vi "main.vi"() -> ()   [LabVIEW 2023] (continued)
      2445  18F106A7   00000004    8        00\tF7\tFF\tFF\tFF\tFF\tFF\tA1\r\n      2445  0CF104A7   00000004    8        F0\t60\t22\tFC\tFF\tFF\tFF\t50\r\n      2444  0CF103A7   00000004    8        17\t1F\t08\t60\tB1\t1F\t08\t50\r\n      2444  0CF102A7   00000004    8        30\t75\tE0\t2E\t80\tFF\tFF\tFD\r\n      2443  0C3C4D4A   00000004    8        BE\tFF\tFF\t7F\t18\tFF\tFF\t50\r\n      2443  0CF101A7   00000004    8        68\t00\t97\tCC\t00\t16\t39\t94\r\n      2442  18F120F0   00000004    8        2B\t75\t60\tB1\tB0\t01\tFF\tFF\r\n      2441  18F11FF0   00000004    8        FF\t3F\t90\t68\t88\t1B\t10\t0C\r\n      2462  1FFFFFFF   00000004    8        00\t20\tFF\tFF\tFF\tFF\tFF\tFF\r\n      2452  1FFFFFFF   00000004    8        00\t20\tFF\tFF\tFF\tFF\tFF\tFF\r\n      2447  1FFFFFFF   00000004    8        00\t20\tFF\tFF\tFF\tFF\tFF\tFF\r\n      2446  18F121F0   00000004    8        09\t19\t00\t00\tFF\tFF\tB0\t01\r\n      2445  18F106A7   00000004    8        00\tF7\tFF\tFF\tFF\tFF\tFF\tA1\r\n      2445  0CF104A7   00000004    8        F0\t60\t22\tFC\tFF\tFF\tFF\t50\r\n      2444  0CF103A7   00000004    8        17\t1F\t08\t60\tB1\t1F\t08\t50\r\n      2444  0CF102A7   00000004    8        30\t75\tE0\t2E\t80\tFF\tFF\tFD\r\n      2443  0C3C4D4A   00000004    8        BE\tFF\tFF\t7F\t18\tFF\tFF\t50\r\n      2443  0CF101A7   00000004    8        68\t00\t97\tCC\t00\t16\t39\t94\r\n      2442  18F120F0   00000004    8        2B\t75\t60\tB1\tB0\t01\tFF\tFF\r\n      2463  0CF101A7   00000004    8        68\t00\t97\tCC\t00\t16\t39\t95\r\n      2462  1FFFFFFF   00000004    8        00\t20\tFF\tFF\tFF\tFF\tFF\tFF\r\n      2452  1FFFFFFF   00000004    8        00\t20\tFF\tFF\tFF\tFF\tFF\tFF\r\n      2447  1FFFFFFF   00000004    8        00\t20\tFF\tFF\tFF\tFF\tFF\tFF\r\n      2446  18F121F0   00000004    8        09\t19\t00\t00\tFF\tFF\tB0\t01\r\n      2445  18F106A7   00000004    8        00\tF7\tFF\tFF\tFF\tFF\tFF\tA1\r\n      2445  0CF104A7   00000004    8        F0\t60\t22\tFC\tFF\tFF\tFF\t50\r\n      2444  0CF103A7   00000004    8        17\t1F\t08\t60\tB1\t1F\t08\t50\r\n      2444  0CF102A7   00000004    8        30\t75\tE0\t2E\t80\tFF\tFF\tFD\r\n      2443  0C3C4D4A   00000004    8        BE\tFF\tFF\t7F\t18\tFF\tFF\t50\r\n      2443  0CF101A7   00000004    8        68\t00\t97\tCC\t00\t16\t39\t94\r\n      2463  0CF102A7   00000004    8        30\t75\tE0\t2E\t80\tFF\tFF\tFD\r\n      2463  0CF101A7   00000004    8        68\t00\t97\tCC\t00\t16\t39\t95\r\n      2462  1FFFFFFF   00000004    8        00\t20\tFF\tFF\tFF\tFF\tFF\tFF\r\n      2452  1FFFFFFF   00000004    8        00\t20\tFF\tFF\tFF\tFF\tFF\tFF\r\n      2447  1FFFFFFF   00000004    8        00\t20\tFF\tFF\tFF\tFF\tFF\tFF\r\n      2446  18F121F0   00000004    8        09\t19\t00\t00\tFF\tFF\tB0\t01\r\n      2445  18F106A7   00000004    8        00\tF7\tFF\tFF\tFF\tFF\tFF\tA1\r\n      2445  0CF104A7   00000004    8        F0\t60\t22\tFC\tFF\tFF\tFF\t50\r\n      2444  0CF103A7   00000004    8        17\t1F\t08\t60\tB1\t1F\t08\t50\r\n      2444  0CF102A7   00000004    8        30\t75\tE0\t2E\t80\tFF\tFF\tFD\r\n      2443  0C3C4D4A   00000004    8        BE\tFF\tFF\t7F\t18\tFF\tFF\t50\r\n      2472  1FFFFFFF   00000004    8        00\t20\tFF\tFF\tFF\tFF\tFF\tFF\r\n      2463  0CF102A7   00000004    8        30\t75\tE0\t2E\t80\tFF\tFF\tFD\r\n      2463  0CF101A7   00000004    8        68\t00\t97\tCC\t00\t16\t39\t95\r\n      2462  1FFFFFFF   00000004    8        00\t20\tFF\tFF\tFF\tFF\tFF\tFF\r\n      2452  1FFFFFFF   00000004    8        00\t20\tFF\tFF\tFF\tFF\tFF\tFF\r\n      2447  1FFFFFFF   00000004    8        00\t20\tFF\tFF\tFF\tFF\tFF\tFF\r\n      2446  18F121F0   00000004    8        09\t19\t00\t00\tFF\tFF\tB0\t01\r\n      2445  18F106A7   00000004    8        00\tF7\tFF\tFF\tFF\tFF\tFF\tA1\r\n      2445  0CF104A7   00000004    8        F0\t60\t22\tFC\tFF\tFF\tFF\t50\r\n      2444  0CF103A7   00000004    8        17\t1F\t08\t60\tB1\t1F\t08\t50\r\n      2444  0CF102A7   00000004    8        30\t75\tE0\t2E\t80\tFF\tFF\tFD\r\n      2482  1FFFFFFF   00000004    8        00\t00\tFF\tFF\tFF\tFF\tFF\tFF\r\n      2472  1FFFFFFF   00000004    8        00\t20\tFF\tFF\tFF\tFF\tFF\tFF\r\n      2463  0CF102A7   00000004    8        30\t75\tE0\t2E\t80\tFF\tFF\tFD\r\n      2463  0CF101A7   00000004    8        68\t00\t97\tCC\t00\t16\t39\t95\r\n      2462  1FFFFFFF   00000004    8        00\t20\tFF\tFF\tFF\tFF\tFF\tFF\r\n      2452  1FFFFFFF   00000004    8        00\t20\tFF\tFF\tFF\tFF\tFF\tFF\r\n      2447  1FFFFFFF   00000004    8        00\t20\tFF\tFF\tFF\tFF\tFF\tFF\r\n      2446  18F121F0   00000004    8        09\t19\t00\t00\tFF\tFF\tB0\t01\r\n      2445  18F106A7   00000004    8        00\tF7\tFF\tFF\tFF\tFF\tFF\tA1\r\n      2445  0CF104A7   00000004    8        F0\t60\t22\tFC\tFF\tFF\tFF\t50\r\n      2444  0CF103A7   00000004    8        17\t1F\t08\t60\tB1\t1F\t08\t50\r\n      2483  0CF101A7   00000004    8        68\t00\t97\tCC\t00\t16\t39\t96\r\n      2482  1FFFFFFF   00000004    8        00\t00\tFF\tFF\tFF\tFF\tFF\tFF\r\n      2472  1FFFFFFF   00000004    8        00\t20\tFF\tFF\tFF\tFF\tFF\tFF\r\n      2463  0CF102A7   00000004    8        30\t75\tE0\t2E\t80\tFF\tFF\tFD\r\n      2463  0CF101A7   00000004    8        68\t00\t97\tCC\t00\t16\t39\t95\r\n      2462  1FFFFFFF   00000004    8        00\t20\tFF\tFF\tFF\tFF\tFF\tFF\r\n      2452  1FFFFFFF   00000004    8        00\t20\tFF\tFF\tFF\tFF\tFF\tFF\r\n      2447  1FFFFFFF   00000004    8        00\t20\tFF\tFF\tFF\tFF\tFF\tFF\r\n      2446  18F121F0   00000004    8        09\t19\t00\t00\tFF\tFF\tB0\t01\r\n      2445  18F106A7   00000004    8        00\tF7\tFF\tFF\tFF\tFF\tFF\tA1\r\n      2445  0CF104A7   00000004    8        F0\t60\t22\tFC\tFF\tFF\tFF\t50\r\n      2483  0CF102A7   00000004    8        30\t75\tE0\t2E\t80\tFF\tFF\tFD\r\n      2483  0CF101A7   00000004    8        68\t00\t97\tCC\t00\t16\t39\t96\r\n      2482  1FFFFFFF   00000004    8        00\t00\tFF\tFF\tFF\tFF\tFF\tFF\r\n      2472  1FFFFFFF   00000004    8        00\t20\tFF\tFF\tFF\tFF\tFF\tFF\r\n      2463  0CF102A7   00000004    8        30\t75\tE0\t2E\t80\tFF\tFF\tFD\r\n      2463  0CF101A7   00000004    8        68\t00\t97\tCC\t00\t16\t39\t95\r\n      2462  1FFFFFFF   00000004    8        00\t20\tFF\tFF\tFF\tFF\tFF\tFF\r\n      2452  1FFFFFFF   00000004    8        00\t20\tFF\tFF\tFF\tFF\tFF\tFF\r\n      2447  1FFFFFFF   00000004    8        00\t20\tFF\tFF\tFF\tFF\tFF\tFF\r\n      2446  18F121F0   00000004    8        09\t19\t00\t00\tFF\tFF\tB0\t01\r\n      2445  18F106A7   00000004    8        00\tF7\tFF\tFF\tFF\tFF\tFF\tA1\r\n      2492  1FFFFFFF   00000004    8        00\t20\tFF\tFF\tFF\tFF\tFF\tFF\r\n      2483  0CF102A7   00000004    8        30\t75\tE0\t2E\t80\tFF\tFF\tFD\r\n      2483  0CF101A7   00000004    8        68\t00\t97\tCC\t00\t16\t39\t96\r\n      2482  1FFFFFFF   00000004    8        00\t00\tFF\tFF\tFF\tFF\tFF\tFF\r\n      2472  1FFFFFFF   00000004    8        00\t20\tFF\tFF\tFF\tFF\tFF\tFF\r\n      2463  0CF102A7   00000004    8        30\t75\tE0\t2E\t80\tFF\tFF\tFD\r\n      2463  0CF101A7   00000004    8        68\t00\t97\tCC\t00\t16\t39\t95\r\n      2462  1FFFFFFF   00000004    8        00\t20\tFF\tFF\tFF\tFF\tFF\tFF\r\n      2452  1FFFFFFF   00000004    8        00\t20\tFF\tFF\tFF\tFF\tFF\tFF\r\n      2447  1FFFFFFF   00000004    8        00\t20\tFF\tFF\tFF\tFF\tFF\tFF\r\n      2446  18F121F0   00000004    8        09\t19\t00\t00\tFF\tFF\tB0\t01\r\n      2493  18F106A7   00000004    8        00\tF7\tFF\tFF\tFF\tFF\tFF\tA2\r\n      2492  1FFFFFFF   00000004    8        00\t20\tFF\tFF\tFF\tFF\tFF\tFF\r\n      2483  0CF102A7   00000004    8        30\t75\tE0\t2E\t80\tFF\tFF\tFD\r\n      2483  0CF101A7   00000004    8        68\t00\t97\tCC\t00\t16\t39\t96\r\n      2482  1FFFFFFF   00000004    8        00\t00\tFF\tFF\tFF\tFF\tFF\tFF\r\n      2472  1FFFFFFF   00000004    8        00\t20\tFF\tFF\tFF\tFF\tFF\tFF\r\n      2463  0CF102A7   00000004    8        30\t75\tE0\t2E\t80\tFF\tFF\tFD\r\n      2463  0CF101A7   00000004    8        68\t00\t97\tCC\t00\t16\t39\t95\r\n      2462  1FFFFFFF   00000004    8        00\t20\tFF\tFF\tFF\tFF\tFF\tFF\r\n      2452  1FFFFFFF   00000004    8        00\t20\tFF\tFF\tFF\tFF\tFF\tFF\r\n      2447  1FFFFFFF   00000004    8        00\t20\tFF\tFF\tFF\tFF\tFF\tFF\r\n      2502  1FFFFFFF   00000004    8        00\t00\tFF\tFF\tFF\tFF\tFF\tFF\r\n      2493  18F106A7   00000004    8        00\tF7\tFF\tFF\tFF\tFF\tFF\tA2\r\n      2492  1FFFFFFF   00000004    8        00\t20\tFF\tFF\tFF\tFF\tFF\tFF\r\n      2483  0CF102A7   00000004    8        30\t75\tE0\t2E\t80\tFF\tFF\tFD\r\n      2483  0CF101A7   00000004    8        68\t00\t97\tCC\t00\t16\t39\t96\r\n      2482  1FFFFFFF   00000004    8        00\t00\tFF\tFF\tFF\tFF\tFF\tFF\r\n      2472  1FFFFFFF   00000004    8        00\t20\tFF\tFF\tFF\tFF\tFF\tFF\r\n      2463  0CF102A7   00000004    8        30\t75\tE0\t2E\t80\tFF\tFF\tFD\r\n      2463  0CF101A7   00000004    8        68\t00\t97\tCC\t00\t16\t39\t95\r\n      2462  1FFFFFFF   00000004    8        00\t20\tFF\tFF\tFF\tFF\tFF\tFF\r\n      2452  1FFFFFFF   00000004    8        00\t20\tFF\tFF\tFF\tFF\tFF\tFF\r\n      2503  0CF101A7   00000004    8        68\t00\t97\tCC\t00\t16\t39\t97\r\n      2502  1FFFFFFF   00000004    8        00\t00\tFF\tFF\tFF\tFF\tFF\tFF\r\n      2493  18F106A7   00000004    8        00\tF7\tFF\tFF\tFF\tFF\tFF\tA2\r\n      2492  1FFFFFFF   00000004    8        00\t20\tFF\tFF\tFF\tFF\tFF\tFF\r\n      2483  0CF102A7   00000004    8        30\t75\tE0\t2E\t80\tFF\tFF\tFD\r\n      2483  0CF101A7   00000004    8        68\t00\t97\tCC\t00\t16\t39\t96\r\n      2482  1FFFFFFF   00000004    8        00\t00\tFF\tFF\tFF\tFF\tFF\tFF\r\n      2472  1FFFFFFF   00000004    8        00\t20\tFF\tFF\tFF\tFF\tFF\tFF\r\n      2463  0CF102A7   00000004    8        30\t75\tE0\t2E\t80\tFF\tFF\tFD\r\n      2463  0CF101A7   00000004    8        68\t00\t97\tCC\t00\t16\t39\t95\r\n      2462  1FFFFFFF   00000004    8        00\t20\tFF\tFF\tFF\tFF\tFF\tFF\r\n      2503  0CF102A7   00000004    8        30\t75\tE0\t2E\t80\tFF\tFF\tFD\r\n      2503  0CF101A7   00000004    8        68\t00\t97\tCC\t00\t16\t39\t97\r\n      2502  1FFFFFFF   00000004    8        00\t00\tFF\tFF\tFF\tFF\tFF\tFF\r\n      2493  18F106A7   00000004    8        00\tF7\tFF\tFF\tFF\tFF\tFF\tA2\r\n      2492  1FFFFFFF   00000004    8        00\t20\tFF\tFF\tFF\tFF\tFF\tFF\r\n      2483  0CF102A7   00000004    8        30\t75\tE0\t2E\t80\tFF\tFF\tFD\r\n      2483  0CF101A7   00000004    8        68\t00\t97\tCC\t00\t16\t39\t96\r\n      2482  1FFFFFFF   00000004    8        00\t00\tFF\tFF\tFF\tFF\tFF\tFF\r\n      2472  1FFFFFFF   00000004    8        00\t20\tFF\tFF\tFF\tFF\tFF\tFF\r\n      2463  0CF102A7   00000004    8        30\t75\tE0\t2E\t80\tFF\tFF\tFD\r\n      2463  0CF101A7   00000004    8        68\t00\t97\tCC\t00\t16\t39\t95\r\n      2512  1FFFFFFF   00000004    8        00\t20\tFF\tFF\tFF\tFF\tFF\tFF\r\n      2503  0CF102A7   00000004    8        30\t75\tE0\t2E\t80\tFF\tFF\tFD\r\n      2503  0CF101A7   00000004    8        68\t00\t97\tCC\t00\t16\t39\t97\r\n      2502  1FFFFFFF   00000004    8        00\t00\tFF\tFF\tFF\tFF\tFF\tFF\r\n      2493  18F106A7   00000004    8        00\tF7\tFF\tFF\tFF\tFF\tFF\tA2\r\n      2492  1FFFFFFF   00000004    8        00\t20\tFF\tFF\tFF\tFF\tFF\tFF\r\n      2483  0CF102A7   00000004    8        30\t75\tE0\t2E\t80\tFF\tFF\tFD\r\n      2483  0CF101A7   00000004    8        68\t00\t97\tCC\t00\t16\t39\t96\r\n      2482  1FFFFFFF   00000004    8        00\t00\tFF\tFF\tFF\tFF\tFF\tFF\r\n      2472  1FFFFFFF   00000004    8        00\t20\tFF\tFF\tFF\tFF\tFF\tFF\r\n      2463  0CF102A7   00000004    8        30\t75\tE0\t2E\t80\tFF\tFF\tFD\r\n      2522  1FFFFFFF   00000004    8        00\t00\tFF\tFF\tFF\tFF\tFF\tFF\r\n      2512  1FFFFFFF   00000004    8        00\t20\tFF\tFF\tFF\tFF\tFF\tFF\r\n      2503  0CF102A7   00000004    8        30\t75\tE0\t2E\t80\tFF\tFF\tFD\r\n      2503  0CF101A7   00000004    8        68\t00\t97\tCC\t00\t16\t39\t97\r\n      2502  1FFFFFFF   00000004    8        00\t00\tFF\tFF\tFF\tFF\tFF\tFF\r\n      2493  18F106A7   00000004    8        00\tF7\tFF\tFF\tFF\tFF\tFF\tA2\r\n      2492  1FFFFFFF   00000004    8        00\t20\tFF\tFF\tFF\tFF\tFF\tFF\r\n      2483  0CF102A7   00000004    8        30\t75\tE0\t2E\t80\tFF\tFF\tFD\r\n      2483  0CF101A7   00000004    8        68\t00\t97\tCC\t00\t16\t39\t96\r\n      2482  1FFFFFFF   00000004    8        00\t00\tFF\tFF\tFF\tFF\tFF\tFF\r\n      2472  1FFFFFFF   00000004    8        00\t20\tFF\tFF\tFF\tFF\tFF\tFF\r\n      2523  0CF101A7   00000004    8        68\t00\t97\tCC\t00\t16\t39\t98\r\n      2522  1FFFFFFF   00000004    8        00\t00\tFF\tFF\tFF\tFF\tFF\tFF\r\n      2512  1FFFFFFF   00000004    8        00\t20\tFF\tFF\tFF\tFF\tFF\tFF\r\n      2503  0CF102A7   00000004    8        30\t75\tE0\t2E\t80\tFF\tFF\tFD\r\n      2503  0CF101A7   00000004    8        68\t00\t97\tCC\t00\t16\t39\t97\r\n      2502  1FFFFFFF   00000004    8        00\t00\tFF\tFF\tFF\tFF\tFF\tFF\r\n      2493  18F106A7   00000004    8        00\tF7\tFF\tFF\tFF\tFF\tFF\tA2\r\n      2492  1FFFFFFF   00000004    8        00\t20\tFF\tFF\tFF\tFF\tFF\tFF\r\n      2483  0CF102A7   00000004    8        30\t75\tE0\t2E\t80\tFF\tFF\tFD\r\n      2483  0CF101A7   00000004    8        68\t00\t97\tCC\t00\t16\t39\t96\r\n      2482  1FFFFFFF   00000004    8        00\t00\tFF\tFF\tFF\tFF\tFF\tFF\r\n      2523  0CF102A7   00000004    8        30\t75\tE0\t2E\t80\tFF\tFF\tFD\r\n      2523  0CF101A7   00000004    8        68\t00\t97\tCC\t00\t16\t39\t98\r\n      2522  1FFFFFFF   00000004    8        00\t00\tFF\tFF\tFF\tFF\tFF\tFF\r\n      2512  1FFFFFFF   00000004    8        00\t20\tFF\tFF\tFF\tFF\tFF\tFF\r\n      2503  0CF102A7   00000004    8        30\t75\tE0\t2E\t80\tFF\tFF\tFD\r\n      2503  0CF101A7   00000004    8        68\t00\t97\tCC\t00\t16\t39\t97\r\n      2502  1FFFFFFF   00000004    8        00\t00\tFF\tFF\tFF\tFF\tFF\tFF\r\n      2493  18F106A7   00000004    8        00\tF7\tFF\tFF\tFF\tFF\tFF\tA2\r\n      2492  1FFFFFFF   00000004    8        00\t20\tFF\tFF\tFF\tFF\tFF\tFF\r\n      2483  0CF102A7   00000004    8        30\t75\tE0\t2E\t80\tFF\tFF\tFD\r\n      2483  0CF101A7   00000004    8        68\t00\t97\tCC\t00\t16\t39\t96\r\n      2532  1FFFFFFF   00000004    8        00\t20\tFF\tFF\tFF\tFF\tFF\tFF\r\n      2523  0CF102A7   00000004    8        30\t75\tE0\t2E\t80\tFF\tFF\tFD\r\n      2523  0CF101A7   00000004    8        68\t00\t97\tCC\t00\t16\t39\t98\r\n      2522  1FFFFFFF   00000004    8        00\t00\tFF\tFF\tFF\tFF\tFF\tFF\r\n      2512  1FFFFFFF   00000004    8        00\t20\tFF\tFF\tFF\tFF\tFF\tFF\r\n      2503  0CF102A7   00000004    8        30\t75\tE0\t2E\t80\tFF\tFF\tFD\r\n      2503  0CF101A7   00000004    8        68\t00\t97\tCC\t00\t16\t39\t97\r\n      2502  1FFFFFFF   00000004    8        00\t00\tFF\tFF\tFF\tFF\tFF\tFF\r\n      2493  18F106A7   00000004    8        00\tF7\tFF\tFF\tFF\tFF\tFF\tA2\r\n      2492  1FFFFFFF   00000004    8        00\t20\tFF\tFF\tFF\tFF\tFF\tFF\r\n      2483  0CF102A7   00000004    8        30\t75\tE0\t2E\t80\tFF\tFF\tFD\r\n      2541  18F11FF0   00000004    8        FF\t3F\t90\t68\t88\t1B\t10\t1C\r\n      2532  1FFFFFFF   00000004    8        00\t20\tFF\tFF\tFF\tFF\tFF\tFF\r\n      2523  0CF102A7   00000004    8        30\t75\tE0\t2E\t80\tFF\tFF\tFD\r\n      2523  0CF101A7   00000004    8        68\t00\t97\tCC\t00\t16\t39\t98\r\n      2522  1FFFFFFF   00000004    8        00\t00\tFF\tFF\tFF\tFF\tFF\tFF\r\n      2512  1FFFFFFF   00000004    8        00\t20\tFF\tFF\tFF\tFF\tFF\tFF\r\n      2503  0CF102A7   00000004    8        30\t75\tE0\t2E\t80\tFF\tFF\tFD\r\n      2503  0CF101A7   00000004    8        68\t00\t97\tCC\t00\t16\t39\t97\r\n      2502  1FFFFFFF   00000004    8        00\t00\tFF\tFF\tFF\tFF\tFF\tFF\r\n      2493  18F106A7   00000004    8        00\tF7\tFF\tFF\tFF\tFF\tFF\tA2\r\n      2492  1FFFFFFF   00000004    8        00\t20\tFF\tFF\tFF\tFF\tFF\tFF\r\n      2542  18F120F0   00000004    8        2B\t75\t60\tB1\tB0\t01\tFF\tFF\r\n      2541  18F11FF0   00000004    8        FF\t3F\t90\t68\t88\t1B\t10\t1C\r\n      2532  1FFFFFFF   00000004    8        00\t20\tFF\tFF\tFF\tFF\tFF\tFF\r\n      2523  0CF102A7   00000004    8        30\t75\tE0\t2E\t80\tFF\tFF\tFD\r\n      2523  0CF101A7   00000004    8        68\t00\t97\tCC\t00\t16\t39\t98\r\n      2522  1FFFFFFF   00000004    8        00\t00\tFF\tFF\tFF\tFF\tFF\tFF\r\n      2512  1FFFFFFF   00000004    8        00\t20\tFF\tFF\tFF\tFF\tFF\tFF\r\n      2503  0CF102A7   00000004    8        30\t75\tE0\t2E\t80\tFF\tFF\tFD\r\n      2503  0CF101A7   00000004    8        68\t00\t97\tCC\t00\t16\t39\t97\r\n      2502  1FFFFFFF   00000004    8        00\t00\tFF\tFF\tFF\tFF\tFF\tFF\r\n      2493  18F106A7   00000004    8        00\tF7\tFF\tFF\tFF\tFF\tFF\tA2\r\n      2543  0CF101A7   00000004    8        68\t00\t97\tCC\t00\t16\t39\t99\r\n      2542  18F120F0   00000004    8        2B\t75\t60\tB1\tB0\t01\tFF\tFF\r\n      2541  18F11FF0   00000004    8        FF\t3F\t90\t68\t88\t1B\t10\t1C\r\n      2532  1FFFFFFF   00000004    8        00\t20\tFF\tFF\tFF\tFF\tFF\tFF\r\n      2523  0CF102A7   00000004    8        30\t75\tE0\t2E\t80\tFF\tFF\tFD\r\n      2523  0CF101A7   00000004    8        68\t00\t97\tCC\t00\t16\t39\t98\r\n      2522  1FFFFFFF   00000004    8        00\t00\tFF\tFF\tFF\tFF\tFF\tFF\r\n      2512  1FFFFFFF   00000004    8        00\t20\tFF\tFF\tFF\tFF\tFF\tFF\r\n      2503  0CF102A7   00000004    8        30\t75\tE0\t2E\t80\tFF\tFF\tFD\r\n      2503  0CF101A7   00000004    8        68\t00\t97\tCC\t00\t16\t39\t97\r\n      2502  1FFFFFFF   00000004    8        00\t00\tFF\tFF\tFF\tFF\tFF\tFF\r\n      2543  0C3C4D4A   00000004    8        BE\tFF\tFF\t7F\t18\tFF\tFF\t51\r\n      2543  0CF101A7   00000004    8        68\t00\t97\tCC\t00\t16\t39\t99\r\n      2542  18F120F0   00000004    8        2B\t75\t60\tB1\tB0\t01\tFF\tFF\r\n      2541  18F11FF0   00000004    8        FF\t3F\t90\t68\t88\t1B\t10\t1C\r\n      2532  1FFFFFFF   00000004    8        00\t20\tFF\tFF\tFF\tFF\tFF\tFF\r\n      2523  0CF102A7   00000004    8        30\t75\tE0\t2E\t80\tFF\tFF\tFD\r\n      2523  0CF101A7   00000004    8        68\t00\t97\tCC\t00\t16\t39\t98\r\n      2522  1FFFFFFF   00000004    8        00\t00\tFF\tFF\tFF\tFF\tFF\tFF\r\n      2512  1FFFFFFF   00000004    8        00\t20\tFF\tFF\tFF\tFF\tFF\tFF\r\n      2503  0CF102A7   00000004    8        30\t75\tE0\t2E\t80\tFF\tFF\tFD\r\n      2503  0CF101A7   00000004    8        68\t00\t97\tCC\t00\t16\t39\t97\r\n      2544  0CF102A7   00000004    8        30\t75\tE0\t2E\t80\tFF\tFF\tFD\r\n      2543  0C3C4D4A   00000004    8        BE\tFF\tFF\t7F\t18\tFF\tFF\t51\r\n      2543  0CF101A7   00000004    8        68\t00\t97\tCC\t00\t16\t39\t99\r\n      2542  18F120F0   00000004    8        2B\t75\t60\tB1\tB0\t01\tFF\tFF\r\n      2541  18F11FF0   00000004    8        FF\t3F\t90\t68\t88\t1B\t10\t1C\r\n      2532  1FFFFFFF   00000004    8        00\t20\tFF\tFF\tFF\tFF\tFF\tFF\r\n      2523  0CF102A7   00000004    8        30\t75\tE0\t2E\t80\tFF\tFF\tFD\r\n      2523  0CF101A7   00000004    8        68\t00\t97\tCC\t00\t16\t39\t98\r\n      2522  1FFFFFFF   00000004    8        00\t00\tFF\tFF\tFF\tFF\tFF\tFF\r\n      2512  1FFFFFFF   00000004    8        00\t20\tFF\tFF\tFF\tFF\tFF\tFF\r\n      2503  0CF102A7   00000004    8        30\t75\tE0\t2E\t80\tFF\tFF\tFD\r\n      2544  0CF103A7   00000004    8        17\t1F\t08\t60\tB1\t1F\t08\t51\r\n      2544  0CF102A7   00000004    8        30\t75\tE0\t2E\t80\tFF\tFF\tFD\r\n      2543  0C3C4D4A   00000004    8        BE\tFF\tFF\t7F\t18\tFF\tFF\t51\r\n      2543  0CF101A7   00000004    8        68\t00\t97\tCC\t00\t16\t39\t99\r\n      2542  18F120F0   00000004    8        2B\t75\t60\tB1\tB0\t01\tFF\tFF\r\n      2541  18F11FF0   00000004    8        FF\t3F\t90\t68\t88\t1B\t10\t1C\r\n      2532  1FFFFFFF   00000004    8        00\t20\tFF\tFF\tFF\tFF\tFF\tFF\r\n      2523  0CF102A7   00000004    8        30\t75\tE0\t2E\t80\tFF\tFF\tFD\r\n      2523  0CF101A7   00000004    8        68\t00\t97\tCC\t00\t16\t39\t98\r\n      2522  1FFFFFFF   00000004    8        00\t00\tFF\tFF\tFF\tFF\tFF\tFF\r\n      2512  1FFFFFFF   00000004    8        00\t20\tFF\tFF\tFF\tFF\tFF\tFF\r\n      2545  0CF104A7   00000004    8        F0\t60\t22\tFC\tFF\tFF\tFF\t51\r\n      2544  0CF103A7   00000004    8        17\t1F\t08\t60\tB1\t1F\t08\t51\r\n      2544  0CF102A7   00000004    8        30\t75\tE0\t2E\t80\tFF\tFF\tFD\r\n      2543  0C3C4D4A   00000004    8        BE\tFF\tFF\t7F\t18\tFF\tFF\t51\r\n      2543  0CF101A7   00000004    8        68\t00\t97\tCC\t00\t16\t39\t99\r\n      2542  18F120F0   00000004    8        2B\t75\t60\tB1\tB0\t01\tFF\tFF\r\n      2541  18F11FF0   00000004    8        FF\t3F\t90\t68\t88\t1B\t10\t1C\r\n      2532  1FFFFFFF   00000004    8        00\t20\tFF\tFF\tFF\tFF\tFF\tFF\r\n      2523  0CF102A7   00000004    8        30\t75\tE0\t2E\t80\tFF\tFF\tFD\r\n      2523  0CF101A7   00000004    8        68\t00\t97\tCC\t00\t16\t39\t98\r\n      2522  1FFFFFFF   00000004    8        00\t00\tFF\tFF\tFF\tFF\tFF\tFF\r\n      2545  18F106A7   00000004    8        00\tF7\tFF\tFF\tFF\tFF\tFF\tA3\r\n      2545  0CF104A7   00000004    8        F0\t60\t22\tFC\tFF\tFF\tFF\t51\r\n      2544  0CF103A7   00000004    8        17\t1F\t08\t60\tB1\t1F\t08\t51\r\n      2544  0CF102A7   00000004    8        30\t75\tE0\t2E\t80\tFF\tFF\tFD\r\n      2543  0C3C4D4A   00000004    8        BE\tFF\tFF\t7F\t18\tFF\tFF\t51\r\n      2543  0CF101A7   00000004    8        68\t00\t97\tCC\t00\t16\t39\t99\r\n      2542  18F120F0   00000004    8        2B\t75\t60\tB1\tB0\t01\tFF\tFF\r\n      2541  18F11FF0   00000004    8        FF\t3F\t90\t68\t88\t1B\t10\t1C\r\n      2532  1FFFFFFF   00000004    8        00\t20\tFF\tFF\tFF\tFF\tFF\tFF\r\n      2523  0CF102A7   00000004    8        30\t75\tE0\t2E\t80\tFF\tFF\tFD\r\n      2523  0CF101A7   00000004    8        68\t00\t97\tCC\t00\t16\t39\t98\r\n      2546  18F121F0   00000004    8        09\t19\t00\t00\tFF\tFF\tB0\t01\r\n      2545  18F106A7   00000004    8        00\tF7\tFF\tFF\tFF\tFF\tFF\tA3\r\n      2545  0CF104A7   00000004    8        F0\t60\t22\tFC\tFF\tFF\tFF\t51\r\n      2544  0CF103A7   00000004    8        17\t1F\t08\t60\tB1\t1F\t08\t51\r\n      2544  0CF102A7   00000004    8        30\t75\tE0\t2E\t80\tFF\tFF\tFD\r\n      2543  0C3C4D4A   00000004    8        BE\tFF\tFF\t7F\t18\tFF\tFF\t51\r\n      2543  0CF101A7   00000004    8        68\t00\t97\tCC\t00\t16\t39\t99\r\n      2542  18F120F0   00000004    8        2B\t75\t60\tB1\tB0\t01\tFF\tFF\r\n      2541  18F11FF0   00000004    8        FF\t3F\t90\t68\t88\t1B\t10\t1C\r\n      2532  1FFFFFFF   00000004    8        00\t20\tFF\tFF\tFF\tFF\tFF\tFF\r\n      2523  0CF102A7   00000004    8        30\t75\tE0\t2E\t80\tFF\tFF\tFD\r\n      2547  1FFFFFFF   00000004    8        00\t20\tFF\tFF\tFF\tFF\tFF\tFF\r\n      2546  18F121F0   00000004    8        09\t19\t00\t00\tFF\tFF\tB0\t01\r\n      2545  18F106A7   00000004    8        00\tF7\tFF\tFF\tFF\tFF\tFF\tA3\r\n      2545  0CF104A7   00000004    8        F0\t60\t22\tFC\tFF\tFF\tFF\t51\r\n      2544  0CF103A7   00000004    8        17\t1F\t08\t60\tB1\t1F\t08\t51\r\n      2544  0CF102A7   00000004    8        30\t75\tE0\t2E\t80\tFF\tFF\tFD\r\n      2543  0C3C4D4A   00000004    8        BE\tFF\tFF\t7F\t18\tFF\tFF\t51\r\n      2543  0CF101A7   00000004    8        68\t00\t97\tCC\t00\t16\t39\t99\r\n      2542  18F120F0   00000004    8        2B\t75\t60\tB1\tB0\t01\tFF\tFF\r\n      2541  18F11FF0   00000004    8        FF\t3F\t90\t68\t88\t1B\t10\t1C\r\n      2532  1FFFFFFF   00000004    8        00\t20\tFF\tFF\tFF\tFF\tFF\tFF\r\n      2552  1FFFFFFF   00000004    8        00\t00\tFF\tFF\tFF\tFF\tFF\tFF\r\n      2547  1FFFFFFF   00000004    8        00\t20\tFF\tFF\tFF\tFF\tFF\tFF\r\n      2546  18F121F0   00000004    8        09\t19\t00\t00\tFF\tFF\tB0\t01\r\n      2545  18F106A7   00000004    8        00\tF7\tFF\tFF\tFF\tFF\tFF\tA3\r\n      2545  0CF104A7   00000004    8        F0\t60\t22\tFC\tFF\tFF\tFF\t51\r\n      2544  0CF103A7   00000004    8        17\t1F\t08\t60\tB1\t1F\t08\t51\r\n      2544  0CF102A7   00000004    8        30\t75\tE0\t2E\t80\tFF\tFF\tFD\r\n      2543  0C3C4D4A   00000004    8        BE\tFF\tFF\t7F\t18\tFF\tFF\t51\r\n      2543  0CF101A7   00000004    8        68\t00\t97\tCC\t00\t16\t39\t99\r\n      2542  18F120F0   00000004    8        2B\t75\t60\tB1\tB0\t01\tFF\tFF\r\n      2541  18F11FF0   00000004    8        FF\t3F\t90\t68\t88\t1B\t10\t1C\r\n      2562  1FFFFFFF   00000004    8        00\t00\tFF\tFF\tFF\tFF\tFF\tFF\r\n      2552  1FFFFFFF   00000004    8        00\t00\tFF\tFF\tFF\tFF\tFF\tFF\r\n      2547  1FFFFFFF   00000004    8        00\t20\tFF\tFF\tFF\tFF\tFF\tFF\r\n      2546  18F121F0   00000004    8        09\t19\t00\t00\tFF\tFF\tB0\t01\r\n      2545  18F106A7   00000004    8        00\tF7\tFF\tFF\tFF\tFF\tFF\tA3\r\n      2545  0CF104A7   00000004    8        F0\t60\t22\tFC\tFF\tFF\tFF\t51\r\n      2544  0CF103A7   00000004    8        17\t1F\t08\t60\tB1\t1F\t08\t51\r\n      2544  0CF102A7   00000004    8        30\t75\tE0\t2E\t80\tFF\tFF\tFD\r\n      2543  0C3C4D4A   00000004    8        BE\tFF\tFF\t7F\t18\tFF\tFF\t51\r\n      2543  0CF101A7   00000004    8        68\t00\t97\tCC\t00\t16\t39\t99\r\n      2542  18F120F0   00000004    8        2B\t75\t60\tB1\tB0\t01\tFF\tFF\r\n      2563  0CF101A7   00000004    8        68\t00\t97\tCC\t00\t16\t39\t9A\r\n      2562  1FFFFFFF   00000004    8        00\t00\tFF\tFF\tFF\tFF\tFF\tFF\r\n      2552  1FFFFFFF   00000004    8        00\t00\tFF\tFF\tFF\tFF\tFF\tFF\r\n      2547  1FFFFFFF   00000004    8        00\t20\tFF\tFF\tFF\tFF\tFF\tFF\r\n      2546  18F121F0   00000004    8        09\t19\t00\t00\tFF\tFF\tB0\t01\r\n      2545  18F106A7   00000004    8        00\tF7\tFF\tFF\tFF\tFF\tFF\tA3\r\n      2545  0CF104A7   00000004    8        F0\t60\t22\tFC\tFF\tFF\tFF\t51\r\n      2544  0CF103A7   00000004    8        17\t1F\t08\t60\tB1\t1F\t08\t51\r\n      2544  0CF102A7   00000004    8        30\t75\tE0\t2E\t80\tFF\tFF\tFD\r\n      2543  0C3C4D4A   00000004    8        BE\tFF\tFF\t7F\t18\tFF\tFF\t51\r\n      2543  0CF101A7   00000004    8        68\t00\t97\tCC\t00\t16\t39\t99\r\n      2563  0CF102A7   00000004    8        30\t75\tE0\t2E\t80\tFF\tFF\tFD\r\n      2563  0CF101A7   00000004    8        68\t00\t97\tCC\t00\t16\t39\t9A\r\n      2562  1FFFFFFF   00000004    8        00\t00\tFF\tFF\tFF\tFF\tFF\tFF\r\n      2552  1FFFFFFF   00000004    8        00\t00\tFF\tFF\tFF\tFF\tFF\tFF\r\n      2547  1FFFFFFF   00000004    8        00\t20\tFF\tFF\tFF\tFF\tFF\tFF\r\n      2546  18F121F0   00000004    8        09\t19\t00\t00\tFF\tFF\tB0\t01\r\n      2545  18F106A7   00000004    8        00\tF7\tFF\tFF\tFF\tFF\tFF\tA3\r\n      2545  0CF104A7   00000004    8        F0\t60\t22\tFC\tFF\tFF\tFF\t51\r\n      2544  0CF103A7   00000004    8        17\t1F\t08\t60\tB1\t1F\t08\t51\r\n      2544  0CF102A7   00000004    8        30\t75\tE0\t2E\t80\tFF\tFF\tFD\r\n      2543  0C3C4D4A   00000004    8        BE\tFF\tFF\t7F\t18\tFF\tFF\t51\r\n      2572  1FFFFFFF   00000004    8        00\t00\tFF\tFF\tFF\tFF\tFF\tFF\r\n      2563  0CF102A7   00000004    8        30\t75\tE0\t2E\t80\tFF\tFF\tFD\r\n      2563  0CF101A7   00000004    8        68\t00\t97\tCC\t00\t16\t39\t9A\r\n      2562  1FFFFFFF   00000004    8        00\t00\tFF\tFF\tFF\tFF\tFF\tFF\r\n      2552  1FFFFFFF   00000004    8        00\t00\tFF\tFF\tFF\tFF\tFF\tFF\r\n      2547  1FFFFFFF   00000004    8        00\t20\tFF\tFF\tFF\tFF\tFF\tFF\r\n      2546  18F121F0   00000004    8        09\t19\t00\t00\tFF\tFF\tB0\t01\r\n      2545  18F106A7   00000004    8        00\tF7\tFF\tFF\tFF\tFF\tFF\tA3\r\n      2545  0CF104A7   00000004    8        F0\t60\t22\tFC\tFF\tFF\tFF\t51\r\n      2544  0CF103A7   00000004    8        17\t1F\t08\t60\tB1\t1F\t08\t51\r\n      2544  0CF102A7   00000004    8        30\t75\tE0\t2E\t80\tFF\tFF\tFD\r\n      2582  1FFFFFFF   00000004    8        00\t00\tFF\tFF\tFF\tFF\tFF\tFF\r\n      2572  1FFFFFFF   00000004    8        00\t00\tFF\tFF\tFF\tFF\tFF\tFF\r\n      2563  0CF102A7   00000004    8        30\t75\tE0\t2E\t80\tFF\tFF\tFD\r\n      2563  0CF101A7   00000004    8        68\t00\t97\tCC\t00\t16\t39\t9A\r\n      2562  1FFFFFFF   00000004    8        00\t00\tFF\tFF\tFF\tFF\tFF\tFF\r\n      2552  1FFFFFFF   00000004    8        00\t00\tFF\tFF\tFF\tFF\tFF\tFF\r\n      2547  1FFFFFFF   00000004    8        00\t20\tFF\tFF\tFF\tFF\tFF\tFF\r\n      2546  18F121F0   00000004    8        09\t19\t00\t00\tFF\tFF\tB0\t01\r\n      2545  18F106A7   00000004    8        00\tF7\tFF\tFF\tFF\tFF\tFF\tA3\r\n      2545  0CF104A7   00000004    8        F0\t60\t22\tFC\tFF\tFF\tFF\t51\r\n      2544  0CF103A7   00000004    8        17\t1F\t08\t60\tB1\t1F\t08\t51\r\n      2583  0CF101A7   00000004    8        68\t00\t97\tCC\t00\t16\t39\t9B\r\n      2582  1FFFFFFF   00000004    8        00\t00\tFF\tFF\tFF\tFF\tFF\tFF\r\n      2572  1FFFFFFF   00000004    8        00\t00\tFF\tFF\tFF\tFF\tFF\tFF\r\n      2563  0CF102A7   00000004    8        30\t75\tE0\t2E\t80\tFF\tFF\tFD\r\n      2563  0CF101A7   00000004    8        68\t00\t97\tCC\t00\t16\t39\t9A\r\n      2562  1FFFFFFF   00000004    8        00\t00\tFF\tFF\tFF\tFF\tFF\tFF\r\n      2552  1FFFFFFF   00000004    8        00\t00\tFF\tFF\tFF\tFF\tFF\tFF\r\n      2547  1FFFFFFF   00000004    8        00\t20\tFF\tFF\tFF\tFF\tFF\tFF\r\n      2546  18F121F0   00000004    8        09\t19\t00\t00\tFF\tFF\tB0\t01\r\n      2545  18F106A7   00000004    8        00\tF7\tFF\tFF\tFF\tFF\tFF\tA3\r\n      2545  0CF104A7   00000004    8        F0\t60\t22\tFC\tFF\tFF\tFF\t51\r\n      2583  0CF102A7   00000004    8        30\t75\tE0\t2E\t80\tFF\tFF\tFD\r\n      2583  0CF101A7   00000004    8        68\t00\t97\tCC\t00\t16\t39\t9B\r\n      2582  1FFFFFFF   00000004    8        00\t00\tFF\tFF\tFF\tFF\tFF\tFF\r\n      2572  1FFFFFFF   00000004    8        00\t00\tFF\tFF\tFF\tFF\tFF\tFF\r\n      2563  0CF102A7   00000004    8        30\t75\tE0\t2E\t80\tFF\tFF\tFD\r\n      2563  0CF101A7   00000004    8        68\t00\t97\tCC\t00\t16\t39\t9A\r\n      2562  1FFFFFFF   00000004    8        00\t00\tFF\tFF\tFF\tFF\tFF\tFF\r\n      2552  1FFFFFFF   00000004    8        00\t00\tFF\tFF\tFF\tFF\tFF\tFF\r\n      2547  1FFFFFFF   00000004    8        00\t20\tFF\tFF\tFF\tFF\tFF\tFF\r\n      2546  18F121F0   00000004    8        09\t19\t00\t00\tFF\tFF\tB0\t01\r\n      2545  18F106A7   00000004    8        00\tF7\tFF\tFF\tFF\tFF\tFF\tA3\r\n      2592  1FFFFFFF   00000004    8        00\t00\tFF\tFF\tFF\tFF\tFF\tFF\r\n      2583  0CF102A7   00000004    8        30\t75\tE0\t2E\t80\tFF\tFF\tFD\r\n      2583  0CF101A7   00000004    8        68\t00\t97\tCC\t00\t16\t39\t9B\r\n      2582  1FFFFFFF   00000004    8        00\t00\tFF\tFF\tFF\tFF\tFF\tFF\r\n      2572  1FFFFFFF   00000004    8        00\t00\tFF\tFF\tFF\tFF\tFF\tFF\r\n      2563  0CF102A7   00000004    8        30\t75\tE0\t2E\t80\tFF\tFF\tFD\r\n      2563  0CF101A7   00000004    8        68\t00\t97\tCC\t00\t16\t39\t9A\r\n      2562  1FFFFFFF   00000004    8        00\t00\tFF\tFF\tFF\tFF\tFF\tFF\r\n      2552  1FFFFFFF   00000004    8        00\t00\tFF\tFF\tFF\tFF\tFF\tFF\r\n      2547  1FFFFFFF   00000004    8        00\t20\tFF\tFF\tFF\tFF\tFF\tFF\r\n      2546  18F121F0   00000004    8        09\t19\t00\t00\tFF\tFF\tB0\t01\r\n      2593  18F106A7   00000004    8        00\tF7\tFF\tFF\tFF\tFF\tFF\tA4\r\n      2592  1FFFFFFF   00000004    8        00\t00\tFF\tFF\tFF\tFF\tFF\tFF\r\n      2583  0CF102A7   00000004    8        30\t75\tE0\t2E\t80\tFF\tFF\tFD\r\n      2583  0CF101A7   00000004    8        68\t00\t97\tCC\t00\t16\t39\t9B\r\n      2582  1FFFFFFF   00000004    8        00\t00\tFF\tFF\tFF\tFF\tFF\tFF\r\n      2572  1FFFFFFF   00000004    8        00\t00\tFF\tFF\tFF\tFF\tFF\tFF\r\n      2563  0CF102A7   00000004    8        30\t75\tE0\t2E\t80\tFF\tFF\tFD\r\n      2563  0CF101A7   00000004    8        68\t00\t97\tCC\t00\t16\t39\t9A\r\n      2562  1FFFFFFF   00000004    8        00\t00\tFF\tFF\tFF\tFF\tFF\tFF\r\n      2552  1FFFFFFF   00000004    8        00\t00\tFF\tFF\tFF\tFF\tFF\tFF\r\n      2547  1FFFFFFF   00000004    8        00\t20\tFF\tFF\tFF\tFF\tFF\tFF\r\n      2602  1FFFFFFF   00000004    8        00\t00\tFF\tFF\tFF\tFF\tFF\tFF\r\n      2593  18F106A7   00000004    8        00\tF7\tFF\tFF\tFF\tFF\tFF\tA4\r\n      2592  1FFFFFFF   00000004    8        00\t00\tFF\tFF\tFF\tFF\tFF\tFF\r\n      2583  0CF102A7   00000004    8        30\t75\tE0\t2E\t80\tFF\tFF\tFD\r\n      2583  0CF101A7   00000004    8        68\t00\t97\tCC\t00\t16\t39\t9B\r\n      2582  1FFFFFFF   00000004    8        00\t00\tFF\tFF\tFF\tFF\tFF\tFF\r\n      2572  1FFFFFFF   00000004    8        00\t00\tFF\tFF\tFF\tFF\tFF\tFF\r\n      2563  0CF102A7   00000004    8        30\t75\tE0\t2E\t80\tFF\tFF\tFD\r\n      2563  0CF101A7   00000004    8        68\t00\t97\tCC\t00\t16\t39\t9A\r\n      2562  1FFFFFFF   00000004    8        00\t00\tFF\tFF\tFF\tFF\tFF\tFF\r\n      2552  1FFFFFFF   00000004    8        00\t00\tFF\tFF\tFF\tFF\tFF\tFF\r\n      2603  0CF101A7   00000004    8        68\t00\t97\tCC\t00\t16\t39\t9C\r\n      2602  1FFFFFFF   00000004    8        00\t00\tFF\tFF\tFF\tFF\tFF\tFF\r\n      2593  18F106A7   00000004    8        00\tF7\tFF\tFF\tFF\tFF\tFF\tA4\r\n      2592  1FFFFFFF   00000004    8        00\t00\tFF\tFF\tFF\tFF\tFF\tFF\r\n      2583  0CF102A7   00000004    8        30\t75\tE0\t2E\t80\tFF\tFF\tFD\r\n      2583  0CF101A7   00000004    8        68\t00\t97\tCC\t00\t16\t39\t9B\r\n      2582  1FFFFFFF   00000004    8        00\t00\tFF\tFF\tFF\tFF\tFF\tFF\r\n      2572  1FFFFFFF   00000004    8        00\t00\tFF\tFF\tFF\tFF\tFF\tFF\r\n      2563  0CF102A7   00000004    8        30\t75\tE0\t2E\t80\tFF\tFF\tFD\r\n      2563  0CF101A7   00000004    8        68\t00\t97\tCC\t00\t16\t39\t9A\r\n      2562  1FFFFFFF   00000004    8        00\t00\tFF\tFF\tFF\tFF\tFF\tFF\r\n      2603  0CF102A7   00000004    8        30\t75\tE0\t2E\t80\tFF\tFF\tFD\r\n      2603  0CF101A7   00000004    8        68\t00\t97\tCC\t00\t16\t39\t9C\r\n      2602  1FFFFFFF   00000004    8        00\t00\tFF\tFF\tFF\tFF\tFF\tFF\r\n      2593  18F106A7   00000004    8        00\tF7\tFF\tFF\tFF\tFF\tFF\tA4\r\n      2592  1FFFFFFF   00000004    8        00\t00\tFF\tFF\tFF\tFF\tFF\tFF\r\n      2583  0CF102A7   00000004    8        30\t75\tE0\t2E\t80\tFF\tFF\tFD\r\n      2583  0CF101A7   00000004    8        68\t00\t97\tCC\t00\t16\t39\t9B\r\n      2582  1FFFFFFF   00000004    8        00\t00\tFF\tFF\tFF\tFF\tFF\tFF\r\n      2572  1FFFFFFF   00000004    8        00\t00\tFF\tFF\tFF\tFF\tFF\tFF\r\n      2563  0CF102A7   00000004    8        30\t75\tE0\t2E\t80\tFF\tFF\tFD\r\n      2563  0CF101A7   00000004    8        68\t00\t97\tCC\t00\t16\t39\t9A\r\n      2612  1FFFFFFF   00000004    8        00\t00\tFF\tFF\tFF\tFF\tFF\tFF\r\n      2603  0CF102A7   00000004    8        30\t75\tE0\t2E\t80\tFF\tFF\tFD\r\n      2603  0CF101A7   00000004    8        68\t00\t97\tCC\t00\t16\t39\t9C\r\n      2602  1FFFFFFF   00000004    8        00\t00\tFF\tFF\tFF\tFF\tFF\tFF\r\n      2593  18F106A7   00000004    8        00\tF7\tFF\tFF\tFF\tFF\tFF\tA4\r\n      2592  1FFFFFFF   00000004    8        00\t00\tFF\tFF\tFF\tFF\tFF\tFF\r\n      2583  0CF102A7   00000004    8        30\t75\tE0\t2E\t80\tFF\tFF\tFD\r\n      2583  0CF101A7   00000004    8        68\t00\t97\tCC\t00\t16\t39\t9B\r\n      2582  1FFFFFFF   00000004    8        00\t00\tFF\tFF\tFF\tFF\tFF\tFF\r\n      2572  1FFFFFFF   00000004    8        00\t00\tFF\tFF\tFF\tFF\tFF\tFF\r\n      2563  0CF102A7   00000004    8        30\t75\tE0\t2E\t80\tFF\tFF\tFD\r\n      2622  1FFFFFFF   00000004    8        00\t00\tFF\tFF\tFF\tFF\tFF\tFF\r\n      2612  1FFFFFFF   00000004    8        00\t00\tFF\tFF\tFF\tFF\tFF\tFF\r\n      2603  0CF102A7   00000004    8        30\t75\tE0\t2E\t80\tFF\tFF\tFD\r\n      2603  0CF101A7   00000004    8        68\t00\t97\tCC\t00\t16\t39\t9C\r\n      2602  1FFFFFFF   00000004    8        00\t00\tFF\tFF\tFF\tFF\tFF\tFF\r\n      2593  18F106A7   00000004    8        00\tF7\tFF\tFF\tFF\tFF\tFF\tA4\r\n      2592  1FFFFFFF   00000004    8        00\t00\tFF\tFF\tFF\tFF\tFF\tFF\r\n      2583  0CF102A7   00000004    8        30\t75\tE0\t2E\t80\tFF\tFF\tFD\r\n      2583  0CF101A7   00000004    8        68\t00\t97\tCC\t00\t16\t39\t9B\r\n      2582  1FFFFFFF   00000004    8        00\t00\tFF\tFF\tFF\tFF\tFF\tFF\r\n      2572  1FFFFFFF   00000004    8        00\t00\tFF\tFF\tFF\tFF\tFF\tFF\r\n      2623  0CF101A7   00000004    8        68\t00\t97\tCC\t00\t16\t39\t9D\r\n      2622  1FFFFFFF   00000004    8        00\t00\tFF\tFF\tFF\tFF\tFF\tFF\r\n      2612  1FFFFFFF   00000004    8        00\t00\tFF\tFF\tFF\tFF\tFF\tFF\r\n      2603  0CF102A7   00000004    8        30\t75\tE0\t2E\t80\tFF\tFF\tFD\r\n      2603  0CF101A7   00000004    8        68\t00\t97\tCC\t00\t16\t39\t9C\r\n      2602  1FFFFFFF   00000004    8        00\t00\tFF\tFF\tFF\tFF\tFF\tFF\r\n      2593  18F106A7   00000004    8        00\tF7\tFF\tFF\tFF\tFF\tFF\tA4\r\n      2592  1FFFFFFF   00000004    8        00\t00\tFF\tFF\tFF\tFF\tFF\tFF\r\n      2583  0CF102A7   00000004    8        30\t75\tE0\t2E\t80\tFF\tFF\tFD\r\n      2583  0CF101A7   00000004    8        68\t00\t97\tCC\t00\t16\t39\t9B\r\n      2582  1FFFFFFF   00000004    8        00\t00\tFF\tFF\tFF\tFF\tFF\tFF\r\n      2623  0CF102A7   00000004    8        30\t75\tE0\t2E\t80\tFF\tFF\tFD\r\n      2623  0CF101A7   00000004    8        68\t00\t97\tCC\t00\t16\t39\t9D\r\n      2622  1FFFFFFF   00000004    8        00\t00\tFF\tFF\tFF\tFF\tFF\tFF\r\n      2612  1FFFFFFF   00000004    8        00\t00\tFF\tFF\tFF\tFF\tFF\tFF\r\n      2603  0CF102A7   00000004    8        30\t75\tE0\t2E\t80\tFF\tFF\tFD\r\n      2603  0CF101A7   00000004    8        68\t00\t97\tCC\t00\t16\t39\t9C\r\n      2602  1FFFFFFF   00000004    8        00\t00\tFF\tFF\tFF\tFF\tFF\tFF\r\n      2593  18F106A7   00000004    8        00\tF7\tFF\tFF\tFF\tFF\tFF\tA4\r\n      2592  1FFFFFFF   00000004    8        00\t00\tFF\tFF\tFF\tFF\tFF\tFF\r\n      2583  0CF102A7   00000004    8        30\t75\tE0\t2E\t80\tFF\tFF\tFD\r\n      2583  0CF101A7   00000004    8        68\t00\t97\tCC\t00\t16\t39\t9B\r\n      2632  1FFFFFFF   00000004    8        00\t20\tFF\tFF\tFF\tFF\tFF\tFF\r\n      2623  0CF102A7   00000004    8        30\t75\tE0\t2E\t80\tFF\tFF\tFD\r\n      2623  0CF101A7   00000004    8        68\t00\t97\tCC\t00\t16\t39\t9D\r\n      2622  1FFFFFFF   00000004    8        00\t00\tFF\tFF\tFF\tFF\tFF\tFF\r\n      2612  1FFFFFFF   00000004    8        00\t00\tFF\tFF\tFF\tFF\tFF\tFF\r\n      2603  0CF102A7   00000004    8        30\t75\tE0\t2E\t80\tFF\tFF\tFD\r\n      2603  0CF101A7   00000004    8        68\t00\t97\tCC\t00\t16\t39\t9C\r\n      2602  1FFFFFFF   00000004    8        00\t00\tFF\tFF\tFF\tFF\tFF\tFF\r\n      2593  18F106A7   00000004    8        00\tF7\tFF\tFF\tFF\tFF\tFF\tA4\r\n      2592  1FFFFFFF   00000004    8        00\t00\tFF\tFF\tFF\tFF\tFF\tFF\r\n      2583  0CF102A7   00000004    8        30\t75\tE0\t2E\t80\tFF\tFF\tFD\r\n      2641  18F11FF0   00000004    8        FF\t3F\t90\t68\t88\t1B\t10\t2C\r\n      2632  1FFFFFFF   00000004    8        00\t20\tFF\tFF\tFF\tFF\tFF\tFF\r\n      2623  0CF102A7   00000004    8        30\t75\tE0\t2E\t80\tFF\tFF\tFD\r\n      2623  0CF101A7   00000004    8        68\t00\t97\tCC\t00\t16\t39\t9D\r\n      2622  1FFFFFFF   00000004    8        00\t00\tFF\tFF\tFF\tFF\tFF\tFF\r\n      2612  1FFFFFFF   00000004    8        00\t00\tFF\tFF\tFF\tFF\tFF\tFF\r\n      2603  0CF102A7   00000004    8        30\t75\tE0\t2E\t80\tFF\tFF\tFD\r\n      2603  0CF101A7   00000004    8        68\t00\t97\tCC\t00\t16\t39\t9C\r\n      2602  1FFFFFFF   00000004    8        00\t00\tFF\tFF\tFF\tFF\tFF\tFF\r\n      2593  18F106A7   00000004    8        00\tF7\tFF\tFF\tFF\t
